vi "Drivetrain Controller.vi"(8 "error in":errorcluster) -> ()   [LabVIEW 2016]
doc: "This VI executes continuously carrying out the current operation and responding to updates or new operations. It will often contain the timing or control code that is difficult to place directly in TeleOp. This VI generally opens all sensors and motors and isolates the rest of the robot code from knowing how the operations are carried out."
uses:
  Drivetrain Setpoints.ctl
  Drivetrain Operations.ctl
  <vilib>/Rock Robotics/WPI/SafetyOutput/WPI_SafetyOutputConfigMenu.ctl
  <vilib>/Rock Robotics/SystemInterfaces/DIO/FPGA_DIOPWMChannel.ctl
  <vilib>/Rock Robotics/WPI/RobotDrive/WPI_RobotDriveOpen4MotorWithVictorSP.vi
  <vilib>/Rock Robotics/WPI/RobotDrive/WPI_RobotDriveMecanumDrive_Cartesian.vi
  <vilib>/Rock Robotics/Network Tables/NT Write Boolean.vi
panel:
  out "Motor Values":dbl[](array[numeric])
  out "Current\nCmd":string
  # "Tip: It may be helpful to observe inputs and sensor values.\nYou may also want to display tuning or debugging controls."
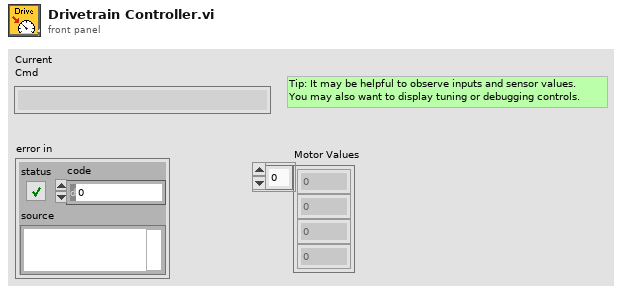
[diagram p1: front panel]
types:
  T1 = typedef "FPGA_DIOPWMChannel.ctl" = enum8{"PWM 0", "PWM 1", "PWM 2", "PWM 3", "PWM 4", "PWM 5", "PWM 6", "PWM 7", "PWM 8", "PWM 9", "PWM MXP 0", "PWM MXP 1", "PWM MXP 2", "PWM MXP 3", "PWM MXP 4", "PWM MXP 5", "PWM MXP 6", "PWM MXP 7", "PWM MXP 8", "PWM MXP 9", "Invalid"}
  T2 = typedef "WPI_SafetyOutputConfigMenu.ctl" = enum16{"Enable", "Disable"}
  T3 = typedef "Drivetrain Setpoints.ctl" = cluster{"Operation":T4, "X Axis":dbl, "Duration":dbl, "Y Axis":dbl, "Rotation":dbl}
  T4 = typedef "Drivetrain Operations.ctl" = enum16{"Reserve", "Default", "Immediate", "Auto"}
  T5 = typedef "WPI_RobotDriveDevRef.ctl" = cluster{"DevStatus":errorcluster, "Motors[]":T6[], "Square Inputs":bool, "Max Output":dbl}
  T6 = typedef "WPI_MotorControlDeviceRef.ctl" = cluster{"DeviceStatus":errorcluster, "Type":T7, "PWM":cluster{"PWM Channel":T1, "DeadBand":T8}, "CAN":cluster{"Device Number":u8, "SetOutput VI Ref":variant, "GetOutput VI Ref":variant, "Enable VI Ref":variant, "Disable VI Ref":variant, "Data":variant}, "Invert":bool}
  T7 = typedef "WPI_MotorControlType.ctl" = enum16{"PWM", "CAN"}
  T8 = typedef "WPI_PWMDeadband.ctl" = cluster{"Name":string, "maxPositivePwm":i32, "minPositivePwm":i32, "centerPwm":i32, "maxNegativePwm":i32, "minNegativePwm":i32, "angularRange":u16}
  T9 = typedef "Command Status Info.ctl" = cluster{"Name":string, "Status":T10, "notifier out":T11}
  T10 = typedef "Completion Status.ctl" = enum16{"Successful", "Aborted", "Incomplete"}
  T11 = typedef "Completion Notifier.ctl" = refnum<notifier>
  T12 = cluster{"Default Command":T3, "Command Timing":cluster{"Start Time (ms)":u32, "Iterations":i32}, "Command Arguments":cluster{"Command Info":T9, "Description":string, "Default Command":T3, "notifier out":refnum<notifier>, "Subsystem Name":string}}
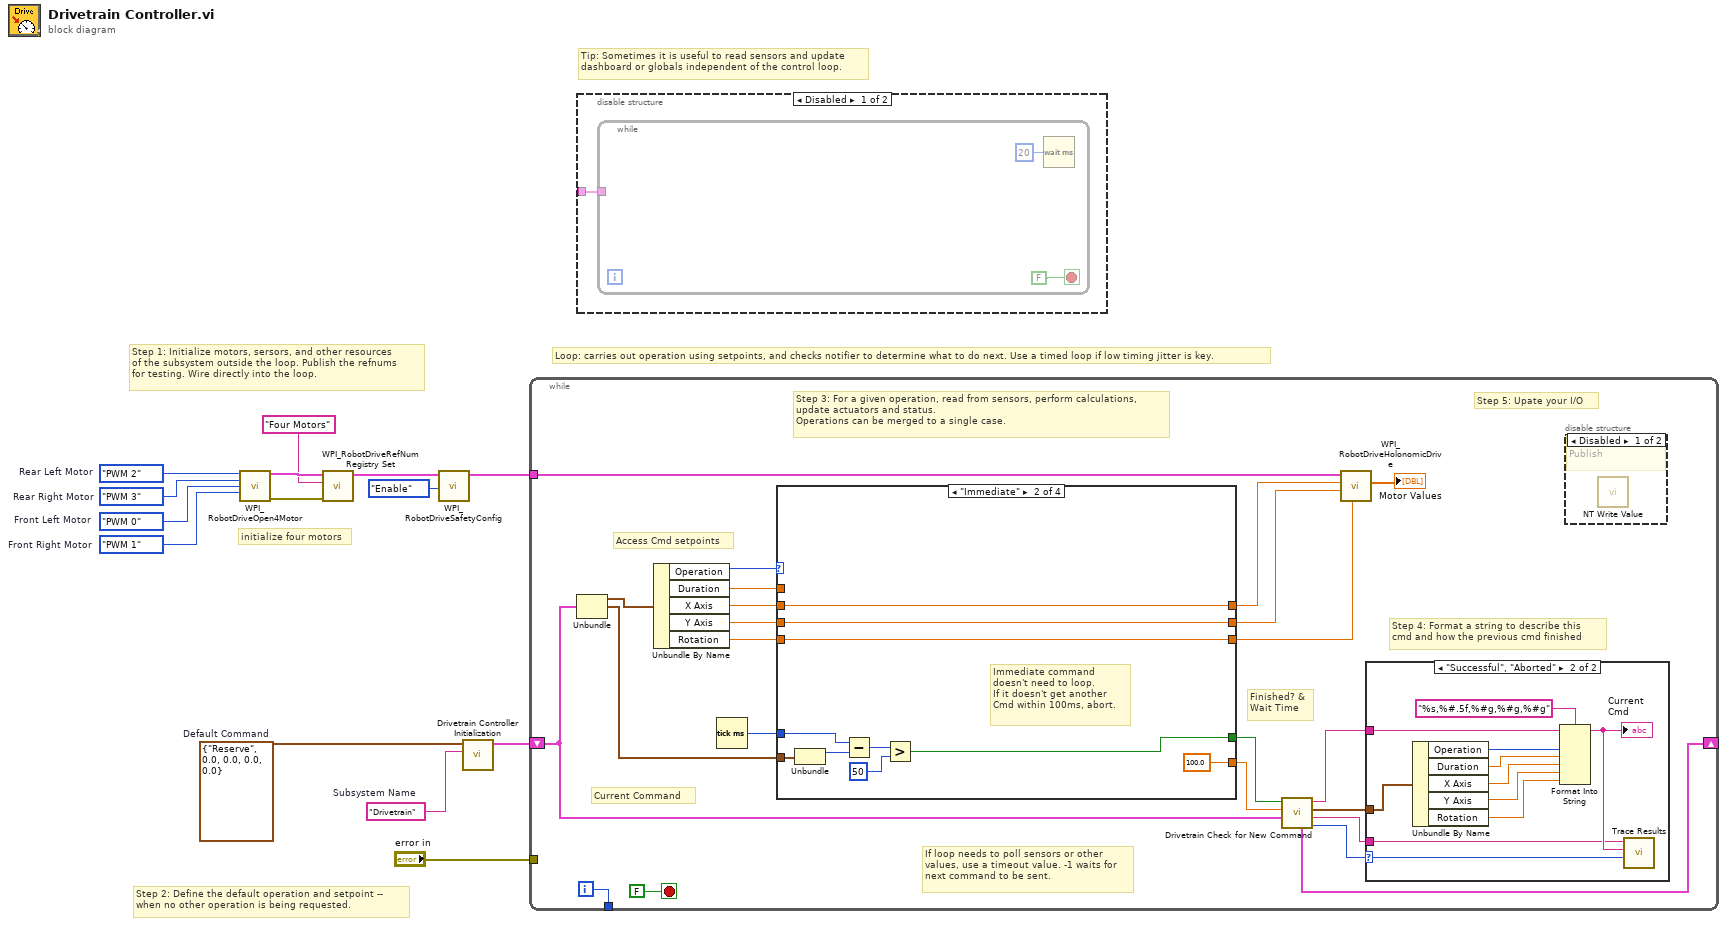
[diagram p0: block diagram]
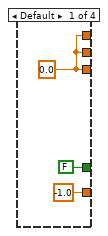
[diagram p5: hidden frame]
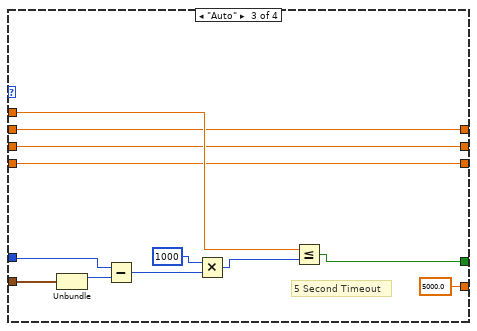
[diagram p6: hidden frame]
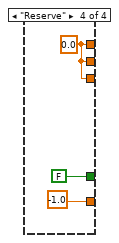
[diagram p7: hidden frame]
diagram:
  w3 = FPGA_DIOPWMChannel."PWM 1"  # Front Right Motor
  w4 = FPGA_DIOPWMChannel."PWM 0"  # Front Left Motor
  w5 = FPGA_DIOPWMChannel."PWM 3"  # Rear Right Motor
  w6 = FPGA_DIOPWMChannel."PWM 2"  # Rear Left Motor
  w11 = T3 {"Operation"=enum."Reserve", "X Axis"=0.0, "Duration"=0.0, "Y Axis"=0.0, "Rotation"=0.0}  # Default Command
  w12 = "Drivetrain"  # Subsystem Name
  # "initialize four motors"
  # "Tip: Sometimes it is useful to read sensors and update\ndashboard or globals independent of the control loop."
  # "Step 2: Define the default operation and setpoint --\nwhen no other operation is being requested."
  # "Step 1: Initialize motors, sersors, and other resources\nof the subsystem outside the loop. Publish the refnums\nfor testing. Wire directly into the loop."
  # "Loop: carries out operation using setpoints, and checks notifier to determine what to do next. Use a timed loop if low timing jitter is key."
  n1 = call-poly <vilib>:"WPI_RobotDriveOpen4Motor.vi"("Rear Left Motor"=w6, "Rear Right Motor"=w5, "Front Left Motor"=w4, "Front Right Motor"=w3) -> ("RobotDriveDevRef"=w10:T5, "error out"=w9:errorcluster)  [unwired: 10 in]
  n2 = call <vilib>:"WPI_RobotDriveRefNum Registry Set.vi"("error in (no error)"=w9, "refnum name"="Four Motors", "RobotDriveDevRef"=w10) -> ("RobotDriveDevRef"=w8:T5)  [unwired: 1 in, 7 out]
  n3 = call <vilib>:"WPI_RobotDriveSafetyConfig.vi"("mode"=WPI_SafetyOutputConfigMenu."Enable", "RobotDriveDevRef"=w8) -> ("RobotDriveDevRef"=w1:T5)  [unwired: 8 in, 1 out]
  n4 = call "Drivetrain Controller Initialization.vi"("Subsystem Name"=w12, "Default Command"=w11) -> ("Command Info"=w13:T12)  [unwired: 9 in]
  n5 = while {
    shift-right: [w28] -> _
    shift-left: w13 -> [w29]
    tunnel: [w36] -> _
    tunnel: "error in" -> [_]
    tunnel: w1 -> [w21]
    i -> [w36]
    stop <- FALSE stop-if-true
    # "If loop needs to poll sensors or other\nvalues, use a timeout value. -1 waits for\nnext command to be sent."
    # "Step 5: Upate your I/O"
    # "Step 4: Format a string to describe this\ncmd and how the previous cmd finished"
    # "Current Command"
    # "Access Cmd setpoints"
    # "Finished? &\nWait Time"
    # "Step 3: For a given operation, read from sensors, perform calculations,\nupdate actuators and status.\nOperations can be merged to a single case."
    n6 = Unbundle(w29) -> ("Default Command"=w35:T3, "Command Timing"=w31:cluster{"Start Time (ms)":u32, "Iterations":i32})  [unwired: 1 out]
    n7 = Unbundle By Name(w35) -> ("Operation"=w34:T4, "Duration"=w33:dbl, "X Axis"=w30:dbl, "Y Axis"=w20:dbl, "Rotation"=w19:dbl)
    n8 = Tick Count (ms)() -> (millisecond timer value=w32:u32)
    n9 = case shown="\"Immediate\"" w34 {
      tunnel: [-1.0 100.0 5000.0 -1.0] -> w26
      tunnel: [FALSE ("ignore previous (F)") w55 w72 FALSE ("ignore previous (F)")] -> w27
      tunnel: w31 -> [_ w57 w68 _]
      tunnel: w33 -> [_ _ w71 _]
      tunnel: w32 -> [_ w56 w69 _]
      tunnel: w30 -> [_ w54 w64 _]
      tunnel: w20 -> [_ w53 w63 _]
      tunnel: w19 -> [_ w52 w62 _]
      tunnel: [w51 w54 w64 w74] -> w18
      tunnel: [w51 w53 w63 w74] -> w17
      tunnel: [w51 w52 w62 w74] -> w16
      frame Default {
        w51 = 0.0 ("Rotation")
      }
      frame "Immediate" {
        # "Immediate command\ndoesn't need to loop.\nIf it doesn't get another\nCmd within 100ms, abort."
        n10 = Unbundle(w57) -> ("Start Time (ms)"=w60:u32)  [unwired: 1 out]
        n11 = Subtract(x=w56, y=w60) -> (x-y=w59:u32)
        n12 = Greater?(x=w59, y=u8 50 ("Left Motor")) -> (0:w55:bool)
      }
      frame "Auto" {
        # "5 Second Timeout"
        n13 = Unbundle(w68) -> ("Start Time (ms)"=w70:u32)  [unwired: 1 out]
        n14 = Subtract(x=w69, y=w70) -> (x-y=w67:u32)
        n15 = Multiply(x=u32 1000, y=w67) -> (x*y=w66:u32)
        n16 = Less Or Equal?(x=w71, y=w66) -> (x <= y?=w72:bool)
      }
      frame "Reserve" {
        w74 = 0.0 ("X Axis")
      }
    }
    n17 = call "Drivetrain Check for New Command.vi"("Current Command"=w29, "Wait time (ms)"=w26, "Finished?"=w27) -> ("Completion"=w22:T10, "Subsystem Name"=w23:string, "Current Command"=w24:T3, "Initial Trace String"=w25:string, "NextCommand"=w28:T12)  [unwired: 4 in]
    n18 = call-poly <vilib>:"WPI_RobotDriveHolonomicDrive.vi"("Rotation"=w16, "Y"=w17, "X"=w18, "RobotDriveDevRef"=w21) -> ("Motor Values"=→"Motor Values":dbl[])  [unwired: 5 in, 2 out]
    n19 = case shown="\"Successful\", \"Aborted\"" w22 {
      selector: w22 -> [_ w48]
      tunnel: w25 -> [_ w46]
      tunnel: w24 -> [_ w47]
      tunnel: w23 -> [_ w44]
      frame "Incomplete", Default {
        # "Continuing current command"
      }
      frame "Successful", "Aborted" {
        # "Report and setup for next command"
        n20 = Unbundle By Name(w47) -> ("Operation"=w43:T4, "Duration"=w42:dbl, "X Axis"=w41:dbl, "Y Axis"=w40:dbl, "Rotation"=w39:dbl)
        n21 = Format Into String(format string="%s,%#.5f,%#g,%#g,%#g", initial string=w46, w43, w42, w41, w40, w39) -> (resulting string=w45:string)  [unwired: 1 in, 1 out]
        "Current\nCmd" <- w45
        n22 = call <vilib>:"Trace Results.vi"("Status of previous command"=w48, "Description"=w45, "Subsystem"=w44) -> ()  [unwired: 9 in]
      }
    }
    n23 = disable-structure shown="Disabled" {
      frame Disabled {
        # "Publish"
        n24 = call-poly <vilib>:"NT Write Value.vi"() -> ()  [unwired: 11 in, 1 out]
      }
      frame Enabled {
      }
    }
  }
  n25 = disable-structure shown="Disabled" {
    disable-tunnel: _ -> [w77 _]
    frame Disabled {
      n26 = while {
        tunnel: w77 -> [_]
        stop <- FALSE stop-if-true
        n27 = Wait (ms)(milliseconds to wait=u32 20) -> ()  [unwired: 1 out]
      }
    }
    frame Enabled {
    }
  }
